vi "Configure Signaling Duplex Mode.vi"(8 "error in (no error)":errorcluster, 9 "Duplex Mode (FDD)":i32(ring) items=["FDD", "TDD"], 10 "Cell Name (\"Cell Name\")":string="Cell Name", 11 "VISA resource name":refnum<visa-resource-name>) -> (0 "error out":errorcluster, 3 "VISA resource name out":refnum<visa-resource-name>)   [LabVIEW 2020, in "Rohde&Schwarz CMWXP NR FR1 Measurement.lvlib"]
doc: "Selects the duplex mode.\n\nAttribute:\nRSCMWXPNRFR1M_ATTR_SIGNALING_DUPLEX_MODE\n\nRemote-control command:\n[CONFigure:]SIGNaling:NRADio:CELL:RFSettings:DMODe"
uses:
  <instrlib>/Rohde&Schwarz CMWXP NR FR1 Measurement/Rohde&Schwarz CMWXP NR FR1 Measurement.lvlib
  <instrlib>/Rohde&Schwarz CMWXP NR FR1 Measurement/Private/rsidr_core.llb/rsidr_core.lvlib
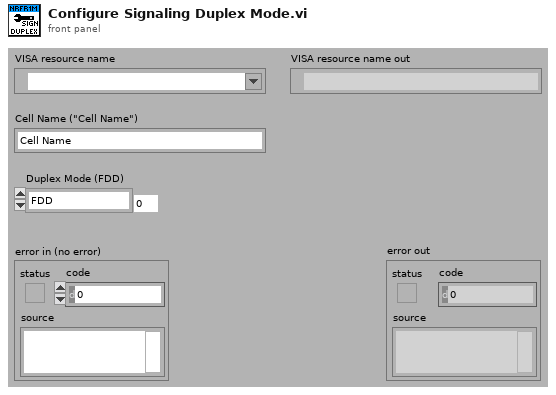
[diagram p1: front panel]
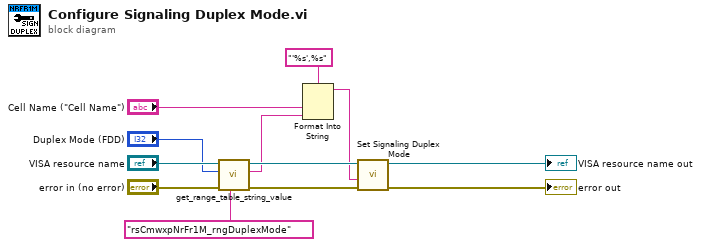
[diagram p0: block diagram]
diagram:
  n1 = call <instrlib>:"get_range_table_string_value.vi"("Range Table ID in"="rsCmwxpNrFr1M_rngDuplexMode", "error in"="error in (no error)", "I32 input"="Duplex Mode (FDD)", "VISA resource name"="VISA resource name") -> ("error out"=w8:errorcluster, "String Value out"=w3:string, "VISA resource name out"=w7:refnum<visa-resource-name>)  [unwired: 5 in]
  n2 = Format Into String(format string="'%s',%s", "Cell Name (\"Cell Name\")", w3) -> (resulting string=w2:string)  [unwired: 2 in, 1 out]
  n3 = call "Set Signaling Duplex Mode"("error in (no error)"=w8, "Signaling Duplex Mode ()"=w2, "instrument handle"=w7) -> ("error out"=→"error out":errorcluster, "instrument handle out"=→"VISA resource name out":refnum<visa-resource-name>)  [unwired: 7 in]
